vi "Git-Extract HTTP Header Value From Keyword.vi"(9 "Key":string, 11 "Header Info":string) -> (1 "Found":bool, 3 "Value":string)   [LabVIEW 2020]
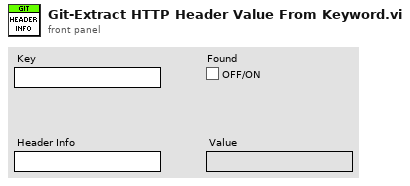
[diagram p1: front panel]
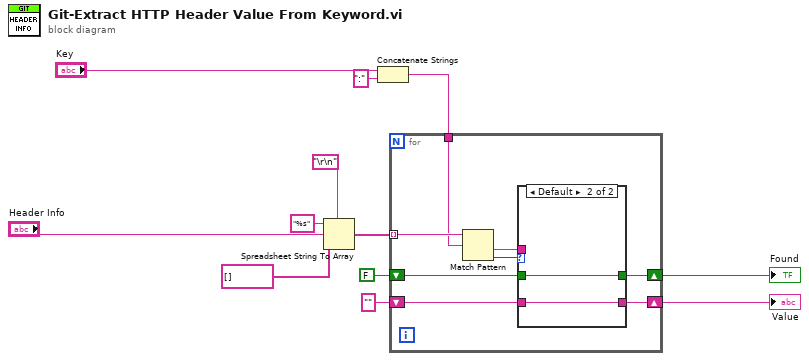
[diagram p0: block diagram]
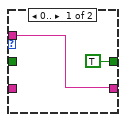
[diagram p2: hidden frame]
diagram:
  n1 = Spreadsheet String To Array(delimiter (Tab)="\r\n", format string="%s", spreadsheet string="Header Info", array type (2D Dbl)=string[] []) -> (array=w5:string[])
  n2 = Concatenate Strings("Key", ":" ("string")) -> (w8:string)
  n3 = for {
    tunnel: w5 -> [w20] mode=indexing
    tunnel: w8 -> [w19]
    shift-right: [w17] -> w10
    shift-left: "" ("after substring") -> [w18]
    shift-right: [w13] -> w12
    shift-left: FALSE -> [w14]
    n4 = Match Pattern(string=w20, regular expression=w19) -> (after substring=w15:string, offset past match=w16:i32)  [unwired: 1 in, 2 out]
    n5 = case shown="Default" w16 {
      tunnel: w18 -> [_ w24]
      tunnel: [w22 w24] -> w17
      tunnel: w15 -> [w22 _]
      tunnel: [TRUE w23] -> w13
      tunnel: w14 -> [_ w23]
      frame 0.. {
      }
      frame Default {
      }
    }
  }
  "Found" <- w12
  "Value" <- w10
